vi "close connection.vi"(8 "error in (no error)":errorcluster, 11 "CEG4500 in":refnum<class "CEG4500.lvclass">) -> (0 "error out":errorcluster, 3 "CEG4500 out":refnum<class "CEG4500.lvclass">)   [LabVIEW 2013, in "CEG4500.lvclass"]
uses:
  CEG4500.lvclass
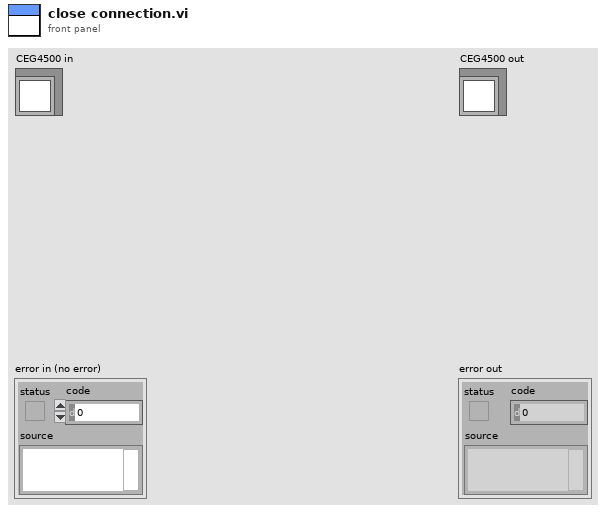
[diagram p1: front panel]
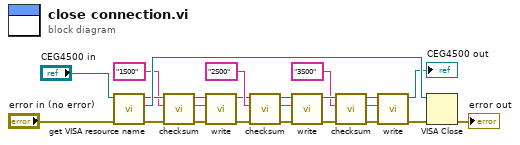
[diagram p0: block diagram]
diagram:
  n1 = call-dynamic "get VISA resource name.vi"("error in (no error)"="error in (no error)", "DeviceInterface (Eingang)"="CEG4500 in") -> ("error out"=w17:errorcluster, "VISA resource name"=w22:refnum<visa-resource-name>, "DeviceInterface (Ausgang)"=w18:refnum<class "CEG4500.lvclass">)  [unwired: 7 in]
  n2 = call-dynamic "checksum.vi"("error in (no error)"=w17, "input"="1S00" ("String to send"), "CEG4500 in"=w18) -> ("error out"=w13:errorcluster, "output"=w15:string, "CEG4500 out"=w14:refnum<class "CEG4500.lvclass">)  [unwired: 6 in]
  n3 = call-dynamic "write.vi"("error in (no error)"=w13, "String to send"=w15, "CEG4500 in"=w14) -> ("error out"=w3:errorcluster, "CEG4500 out"=w6:refnum<class "CEG4500.lvclass">)  [unwired: 7 in]
  n4 = call-dynamic "checksum.vi"("error in (no error)"=w3, "input"="2S00" ("String to send"), "CEG4500 in"=w6) -> ("error out"=w4:errorcluster, "output"=w8:string, "CEG4500 out"=w5:refnum<class "CEG4500.lvclass">)  [unwired: 6 in]
  n5 = call-dynamic "write.vi"("error in (no error)"=w4, "String to send"=w8, "CEG4500 in"=w5) -> ("error out"=w2:errorcluster, "CEG4500 out"=w12:refnum<class "CEG4500.lvclass">)  [unwired: 7 in]
  n6 = call-dynamic "checksum.vi"("error in (no error)"=w2, "input"="3S00" ("String to send"), "CEG4500 in"=w12) -> ("error out"=w1:errorcluster, "output"=w10:string, "CEG4500 out"=w11:refnum<class "CEG4500.lvclass">)  [unwired: 6 in]
  n7 = call-dynamic "write.vi"("error in (no error)"=w1, "String to send"=w10, "CEG4500 in"=w11) -> ("error out"=w19:errorcluster, "CEG4500 out"=→"CEG4500 out":refnum<class "CEG4500.lvclass">)  [unwired: 7 in]
  n8 = VISA Close(VISA resource name=w22, error in (no error)=w19) -> (error out=→"error out":errorcluster)
